vi "Drive Teleop.vi"(11 "Joystick Vals":T1) -> ()   [LabVIEW 2016]
uses:
  Joystick vals.ctl
  <vilib>/Rock Robotics/Network Tables/NT Write Boolean.vi
  <vilib>/Rock Robotics/Network Tables/NT Write Number.vi
panel:
  out "max(x,y)":i32
  in  "Distance (ft)":dbl=6.0 format="%#_13g"
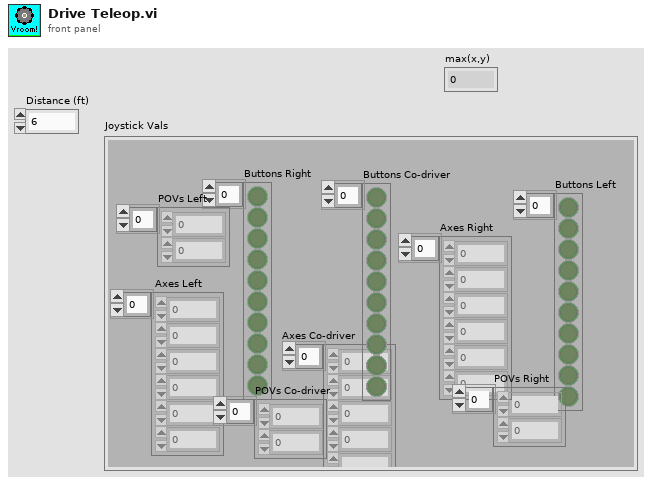
[diagram p1: front panel]
types:
  T1 = typedef "Joystick vals.ctl" = cluster{"Axes Right":dbl[], " Axes Left":dbl[], " Axes Co-driver":dbl[], "Buttons Right":bool[], "Buttons Left":bool[], "Buttons Co-driver":bool[], "POVs Right":i16[], "POVs Left":i16[], "POVs Co-driver":i16[]}
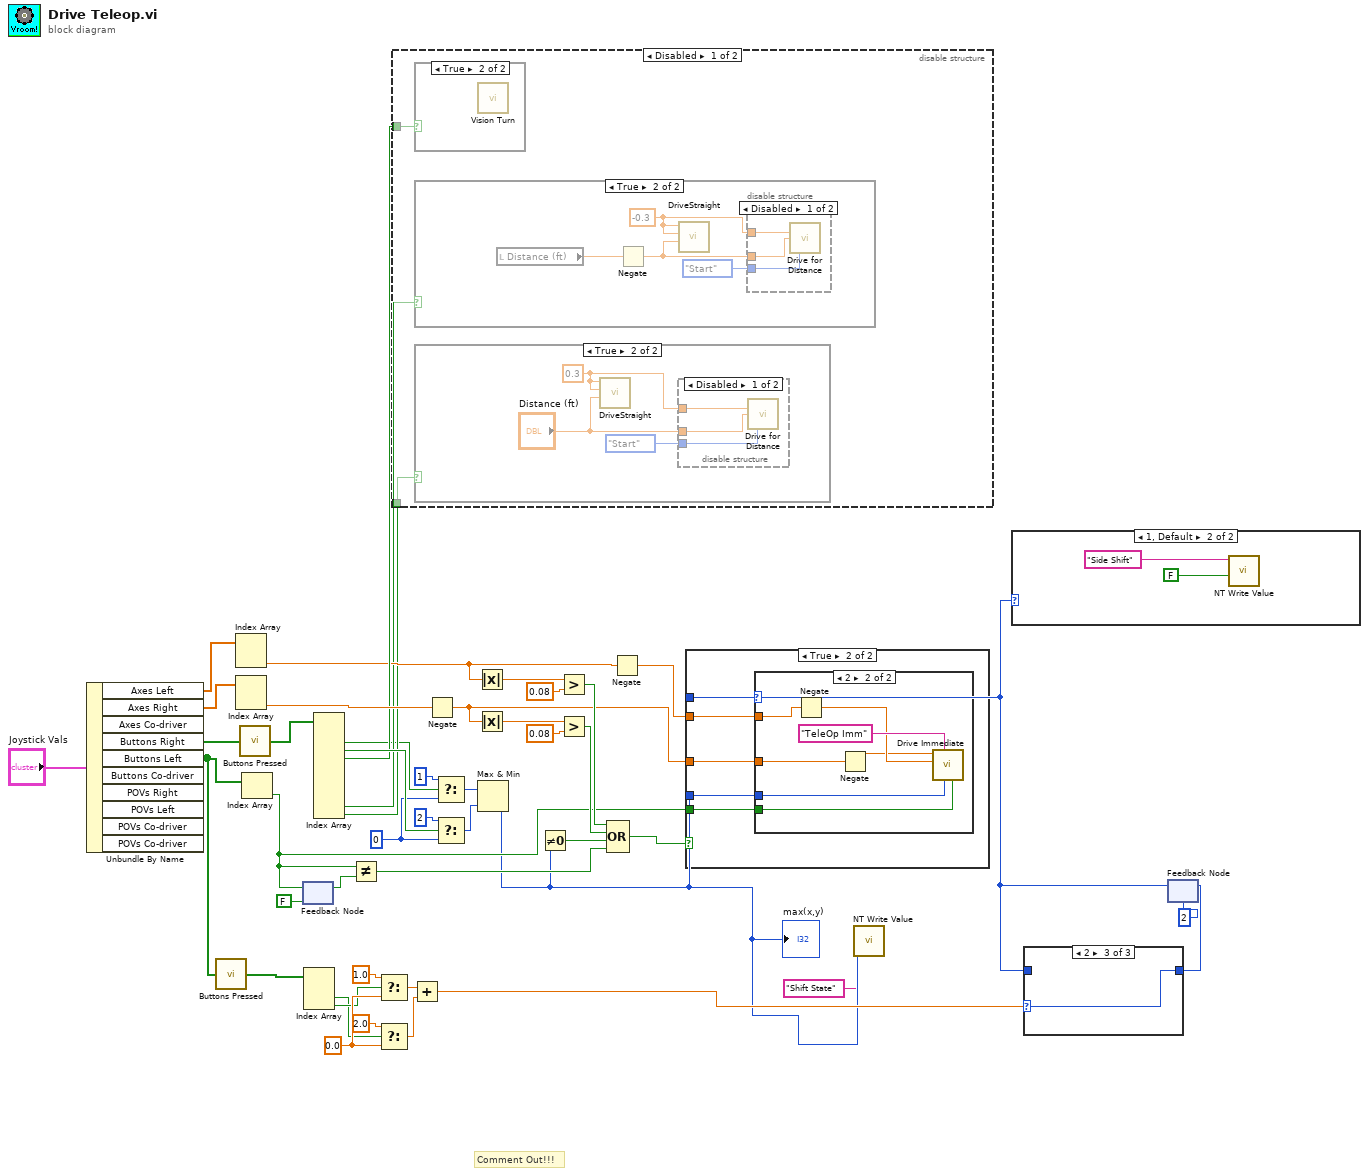
[diagram p0: block diagram]
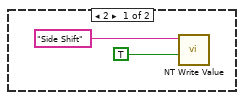
[diagram p8: hidden frame]
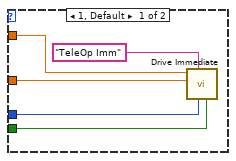
[diagram p12: hidden frame]
diagram:
  w19 = 0.0 ("f")
  w43 = 0
  # "Comment Out!!!"
  n1 = Unbundle By Name("Joystick Vals") -> ("Axes Left"=w29:dbl[], "Axes Right"=w28:dbl[], "Buttons Right"=w23:bool[], "Buttons Left"=w11:bool[])  [unwired: 6 out]
  n2 = call "Buttons Pressed.vi"("Button Values"=w11) -> ("Button Presses"=w21:bool[])
  n3 = Index Array(array=w29) -> (element #2=w26:dbl)  [unwired: 2 in, 1 out]
  n4 = Index Array(array=w28) -> (element #2=w33:dbl)  [unwired: 2 in, 1 out]
  n5 = call "Buttons Pressed.vi"("Button Values"=w23) -> ("Button Presses"=w46:bool[])
  n6 = Index Array(array=w11) -> (element=w7:bool)  [unwired: 1 in]
  n7 = feedback-in #1(w7) -> ()
  n8 = feedback #1(FALSE) -> (w10:bool)
  n9 = Index Array(array=w21) -> (element #2=w13:bool, element #3=w14:bool)  [unwired: 3 in, 1 out]
  n10 = Index Array(array=w46) -> (element #2=w3:bool, element #3=w45:bool, element #4=w27:bool, element #10=w5:bool, element #11=w6:bool)  [unwired: 11 in, 6 out]
  n11 = Not Equal?(x=w7, y=w10) -> (x != y?=w8:bool)
  n12 = Select(t=1.0, s=w14, f=w19) -> (s? t:f=w17:dbl)
  n13 = Select(t=2.0, s=w13, f=w19) -> (s? t:f=w16:dbl)
  n14 = disable-structure shown="Disabled" {
    disable-tunnel: w27 -> [w49 _]
    disable-tunnel: w6 -> [w48 _]
    disable-tunnel: w5 -> [w47 _]
    frame Disabled {
      n15 = case shown="True" w49 {
        frame False {
        }
        frame True {
          n16 = call "Vision Turn.vi"() -> ()  [unwired: 11 in, 1 out]
        }
      }
      n17 = case shown="True" w47 {
        frame False {
        }
        frame True {
          w52 = -0.3 ("speed")
          n18 = local read "Distance (ft)"() -> (w51:dbl)
          n19 = Negate(x=w51) -> (-x=w50:dbl)
          n20 = call "DriveStraight.vi"("Seconds"=w50, "Right Speed"=w52, "Left Speed"=w52) -> ()  [unwired: 7 in, 2 out]
          n21 = disable-structure shown="Disabled" {
            disable-tunnel: w52 -> [w56 _]
            disable-tunnel: w50 -> [w55 _]
            disable-tunnel: enum16{"Start", "Wait"}."Start" ("Synchronication") -> [w54 _]
            frame Disabled {
              n22 = call "Drive for Distance.vi"("speed"=w56, "Distance (ft)"=w55, "Synchronication"=w54) -> ()  [unwired: 12 in, 1 out]
            }
            frame Enabled {
            }
          }
        }
      }
      n23 = case shown="True" w48 {
        frame False {
        }
        frame True {
          w58 = 0.3 ("speed")
          n24 = call "DriveStraight.vi"("Seconds"="Distance (ft)", "Right Speed"=w58, "Left Speed"=w58) -> ()  [unwired: 7 in, 2 out]
          n25 = disable-structure shown="Disabled" {
            disable-tunnel: w58 -> [w62 _]
            disable-tunnel: "Distance (ft)" -> [w61 _]
            disable-tunnel: enum16{"Start", "Wait"}."Start" ("Synchronication") -> [w60 _]
            frame Disabled {
              n26 = call "Drive for Distance.vi"("speed"=w62, "Distance (ft)"=w61, "Synchronication"=w60) -> ()  [unwired: 12 in, 1 out]
            }
            frame Enabled {
            }
          }
        }
      }
    }
    frame Enabled {
    }
  }
  n27 = Add(x=w17, y=w16) -> (x+y=w15:dbl)
  n28 = Negate(x=w33) -> (-x=w24:dbl)
  n29 = Select(t=1, s=w3, f=w43) -> (s? t:f=w41:i32)
  n30 = Select(t=2, s=w45, f=w43) -> (s? t:f=w40:i32)
  n31 = Absolute Value(x=w26) -> (abs(x)=w37:dbl)
  n32 = Absolute Value(x=w24) -> (abs(x)=w34:dbl)
  n33 = Max & Min(x=w41, y=w40) -> (max(x,y)=w2:i32)  [unwired: 1 out]
  "max(x,y)" <- w2
  n34 = Not Equal To 0?(x=w2) -> (x != 0?=w39:bool)
  n35 = Greater?(x=w37, y=0.08) -> (0:w35:bool)
  n36 = Greater?(x=w34, y=0.08) -> (0:w31:bool)
  n37 = Compound Arithmetic op=OR(w35, w31, w39, w8) -> (w38:bool)
  n38 = Negate(x=w26) -> (-x=w25:dbl)
  n39 = call-poly <vilib>:"NT Write Value.vi"("Numeric"=w2, "Name"="Shift State") -> ()  [unwired: 9 in, 1 out]
  n40 = feedback #2(2) -> (w12:i32)
  n41 = case shown="True" w38 {
    tunnel: w2 -> [_ w67]
    tunnel: w24 -> [_ w65]
    tunnel: w25 -> [_ w66]
    tunnel: w12 -> [_ w64]
    tunnel: w7 -> [_ w63]
    frame False {
    }
    frame True {
      n42 = case shown="2" w64 {
        tunnel: w67 -> [w71 w78]
        tunnel: w66 -> [w70 w77]
        tunnel: w65 -> [w69 w76]
        tunnel: w63 -> [w68 w73]
        frame 1, Default {
          n43 = call "Drive Immediate.vi"("Brake"=w68, "Shift"=w71, "Description"="TeleOp Imm", "Right Setpoint"=w69, "Left Setpoint"=w70) -> ()  [unwired: 6 in, 1 out]
        }
        frame 2 {
          n44 = Negate(x=w77) -> (-x=w75:dbl)
          n45 = Negate(x=w76) -> (-x=w74:dbl)
          n46 = call "Drive Immediate.vi"("Brake"=w73, "Shift"=w78, "Description"="TeleOp Imm", "Right Setpoint"=w75, "Left Setpoint"=w74) -> ()  [unwired: 6 in, 1 out]
        }
      }
    }
  }
  n47 = case shown="1, Default" w12 {
    frame 2 {
      n48 = call-poly <vilib>:"NT Write Value.vi"("Boolean"=TRUE, "Name"="Side Shift") -> ()  [unwired: 9 in, 1 out]
    }
    frame 1, Default {
      n49 = call-poly <vilib>:"NT Write Value.vi"("Boolean"=FALSE, "Name"="Side Shift") -> ()  [unwired: 9 in, 1 out]
    }
  }
  n50 = case shown="2" w15 {
    selector: w15 -> [_ w85 w86]
    tunnel: w12 -> [w84 _ _]
    tunnel: [w84 w85 w86] -> w4
    frame 0, Default {
    }
    frame 1 {
    }
    frame 2 {
    }
  }
  n51 = feedback-in #2(w4) -> ()
